vi "Actor Core.vi"(8 "error in":errorcluster, 11 "Logger Mananger in":refnum<class "Logger Mananger.lvclass">) -> (0 "error out":errorcluster, 3 "Actor out":refnum<class "Actor.lvclass">)   [LabVIEW 2020, in "Logging.lvlib" / "Logger Mananger.lvclass"]
doc: "(<B>Filename</B>: Actor Framework.lvlib:Actor.lvclass:Actor Core.vi)\n\nReceives messages to the actor, reacts to them, and initiates any error handling that may shut the actor down.\n\nDescendant classes may override this VI to append parallel tasks for the actor to complete while it handles messages. Overrides use the Call Parent Class Method node."
uses:
  Logger Mananger.lvclass
  <vilib>/ActorFramework/Actor/Actor.lvclass
  Global Log.vi
  Logging.lvlib
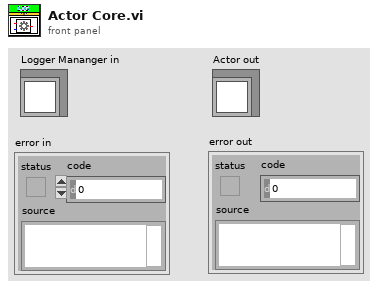
[diagram p1: front panel]
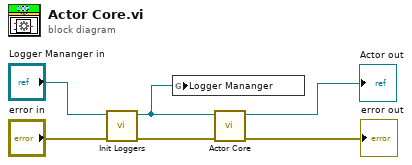
[diagram p0: block diagram]
diagram:
  n1 = call "Init Loggers.vi"("error in (no error)"="error in", "Logger Mananger in"="Logger Mananger in") -> ("error out"=w2:errorcluster, "Logger Mananger out"=w1:refnum<class "Logger Mananger.lvclass">)  [unwired: 8 in]
  n2 = global write "Global Log.vi" "Logger Mananger"(w1) -> ()
  n3 = call-parent "Actor Core.vi"("error in"=w2, "Actor in"=w1) -> ("error out"=→"error out":errorcluster, "Actor out"=→"Actor out":refnum<class "Actor.lvclass">)  [unwired: 8 in]
